vi "Go_Inicial.vi"(0 "task/channels in":refnum<k21>, 1 "Start_A":dbl caption="Ángulo inicial" min=-5.0 max=5.0 step=0.05, 2 "Fi":dbl=0.01 caption="Desfase ángulo" min=-0.8 max=0.8 step=0.01, 5 "Error In":errorcluster, 7 "ms to wait":u32=20) -> (19 "Error Out":errorcluster)   [LabVIEW 2016]
doc: "Va a la posición inicial del recorrido\n\n----\nDesarrollado por:\nIng. Jhony Turizo\nFebrero 2017"
uses:
  <vilib>/DAQmx/write.llb/DAQmx Write (Analog DBL 1Chan 1Samp).vi
  <vilib>/DAQmx/miscellaneous.llb/DAQmx Fill In Error Info.vi
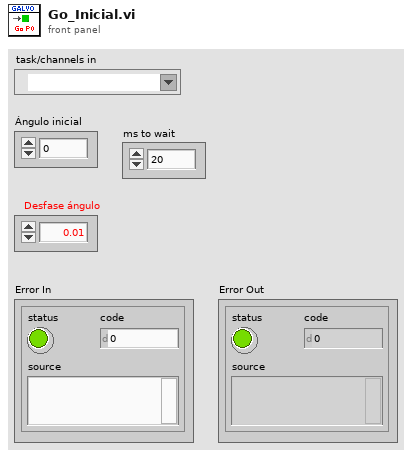
[diagram p1: front panel]
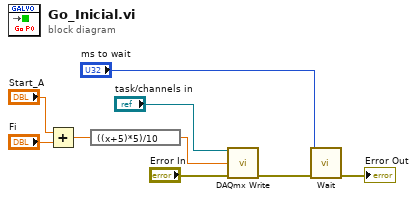
[diagram p0: block diagram]
diagram:
  n1 = Add(x="Start_A", y="Fi") -> (x+y=w5:dbl)
  n2 = expression code="((x+5)*5)/10"(w5) -> (w7:dbl)
  n3 = call-poly <vilib>:"DAQmx Write.vi"("task/channels in"="task/channels in", "data"=w7, "error in"="Error In") -> ("error out"=w3:errorcluster)  [unwired: 10 in, 2 out]
  n4 = call "Wait.vi"("Error In"=w3, "ms to wait"="ms to wait") -> ("Error Out"=→"Error Out":errorcluster)  [unwired: 9 in]
